vi "Output Trigger Query.vi"(8 "error in":errorcluster, 10 "Trigger Output":i32(ring) items=["TTL0", "TTL1", "TTL2", "TTL3", "TTL4", "TTL5", "TTL6", "TTL7", "ECL0", "ECL1"], 11 "Instrument Handle In":i32) -> (0 "error out":errorcluster, 1 "Source":i32, 2 "State":i32, 3 "Instrument Handle Out":i32, 4 "Polarity":i32)   [LabVIEW 8.6, in "ZTScopeM.lvlib"]
doc: "Query the selected bus trigger's configuration."
uses:
  ZTScopeM.lvlib
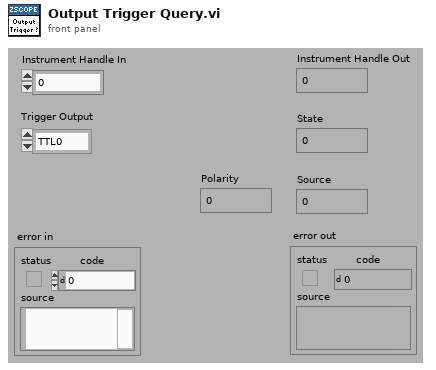
[diagram p1: front panel]
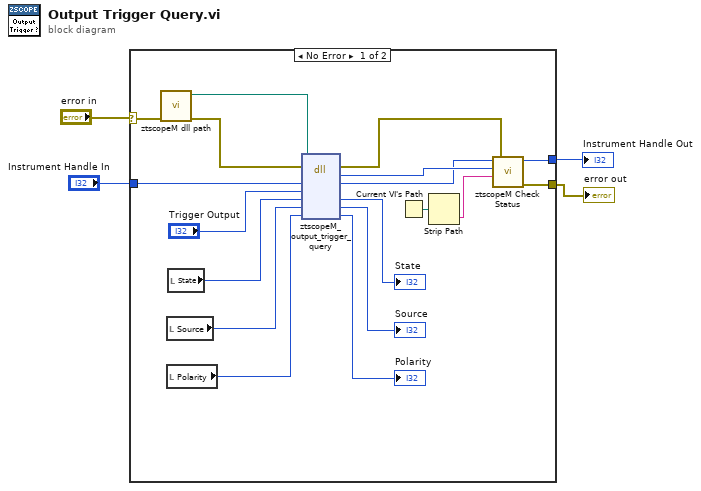
[diagram p0: block diagram]
diagram:
  n1 = case shown="No Error" "error in" {
    selector: "error in" -> [w8 w24]
    tunnel: [w9 w24] -> w1
    tunnel: "Instrument Handle In" -> [w22 w23]
    tunnel: [w10 w23] -> w3
    frame #0 {
      n2 = call "ztscopeM dll path.vi"("error in (no error)"=w8) -> ("error out"=w6:errorcluster, "<instrument>.dll path"=w7:path)  [unwired: 9 in]
      n3 = local read "Source"() -> (w18:i32)
      n4 = local read "Polarity"() -> (w16:i32)
      n5 = local read "State"() -> (w20:i32)
      n6 = dll-call lib="C:/Program Files (x86)/National Instruments/LabVIEW 2013/instr.lib/ztscopem/ztscopeM.dll" fn="ztscopeM_output_trigger_query"(path in=w7, error in=w6, "instrumentHandle"=w22, "triggerOutput"="Trigger Output", "state"=w20, "source"=w18, "polarity"=w16) -> (error out=w5:errorcluster, w12:i32, "instrumentHandle"=w11:i32, "state"=→"State":i32, "source"=→"Source":i32, "polarity"=→"Polarity":i32)  [unwired: 2 in, 1 out]
      n7 = Current VI's Path() -> (path=w14:path)
      n8 = Strip Path(path=w14) -> (name=w13:string)  [unwired: 1 out]
      n9 = call "ztscopeM Check Status.vi"("error in"=w5, "name of VI"=w13, "status (return code)"=w12, "instrument handle in"=w11) -> ("error out"=w9:errorcluster, "instrument handle out"=w10:i32)  [unwired: 2 in]
    }
    frame #1 {
    }
  }
  "Instrument Handle Out" <- w3
  "error out" <- w1
